vi "Template - P-C StartStop.vi"(7 "Selector":enum16{"Start C-P ", "Clear C-P"}(ring), 8 "error in":errorcluster) -> (0 "error out":errorcluster)   [LabVIEW 2012]
uses:
  Navistar Library/Controls/TypeDef - UEvent Selector(Standard).ctl
  Navistar Library/Controls/TypeDef - Queue Selector(Standard).ctl
  Navistar Library/Controls/TypeDef_Error_Command_enum.ctl
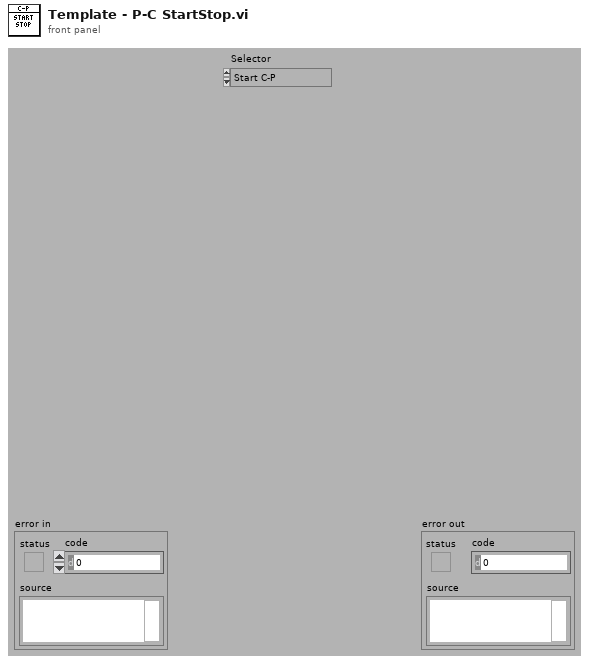
[diagram p1: front panel]
types:
  T1 = typedef "TypeDef_Error_Command_enum.ctl" = enum16{"Init", "Check", "Report"}
  T2 = typedef "TypeDef - UEvent Selector(Standard).ctl" = enum16{"Create UEvent", "Get UEvent Ref", "Clear UEvent", "Reset UEvent", "Generate U Event"}
  T3 = typedef "TypeDef - Queue Selector(Standard).ctl" = enum16{"Create Q", "EnQ", "EnQ at the Opposite", "Flush Q", "Get Q Ref", "Clear Q", "Reset Q"}
  T4 = typedef "TypeDef - Template - UEvent Ref.ctl" = refnum<user-event>
  T5 = typedef "TypeDef - Template - Q1 Ref.ctl" = refnum<queue>
  T6 = typedef "TypeDef - Template - Q2 Ref.ctl" = refnum<queue>
  T7 = cluster{"Q1 Ref":T5, "Q2 Ref":T6, "U-Event Refnum":T4}
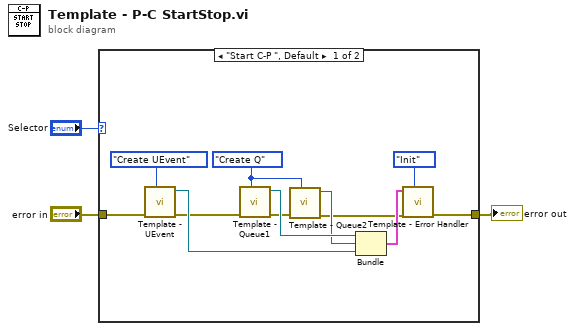
[diagram p0: block diagram]
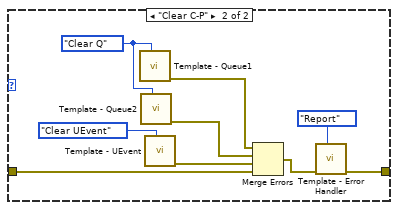
[diagram p2: hidden frame]
diagram:
  n1 = case shown="\"Start C-P \", Default" "Selector" {
    tunnel: "error in" -> [w6 w24]
    tunnel: [w14 w19] -> w2
    frame "Start C-P ", Default {
      w10 = TypeDef_-_Queue_Selector(Standard)."Create Q" ("Queue Selector")
      n2 = call "Template - UEvent.vi"("Event Selector"=TypeDef_-_UEvent_Selector(Standard)."Create UEvent", "error in (no error)"=w6) -> ("error out"=w5:errorcluster, "U-Event Refnum"=w8:T4)  [unwired: 7 in, 1 out]
      n3 = call "Template - Queue1.vi"("Queue Selector"=w10, "error in (no error)"=w5) -> ("error out"=w11:errorcluster, "Q1 Ref"=w12:T5)  [unwired: 7 in, 1 out]
      n4 = call "Template - Queue2.vi"("Queue Selector"=w10, "error in (no error)"=w11) -> ("error out"=w4:errorcluster, "Q2 Ref"=w9:T6)  [unwired: 7 in, 1 out]
      n5 = Bundle("Q1 Ref"=w12, "Q2 Ref"=w9, "U-Event Refnum"=w8) -> (w7:T7)  [unwired: 1 in]
      n6 = call "Template - Error Handler.vi"("Command (Check for Error)"=TypeDef_Error_Command_enum."Init", "error in (no error)"=w4, "QU Ref cluster"=w7) -> ("error out"=w14:errorcluster)  [unwired: 8 in]
    }
    frame "Clear C-P" {
      w17 = TypeDef_-_Queue_Selector(Standard)."Clear Q" ("Queue Selector")
      n7 = call "Template - Queue1.vi"("Queue Selector"=w17) -> ("error out"=w22:errorcluster)  [unwired: 8 in, 2 out]
      n8 = call "Template - Queue2.vi"("Queue Selector"=w17) -> ("error out"=w16:errorcluster)  [unwired: 8 in, 2 out]
      n9 = call "Template - UEvent.vi"("Event Selector"=TypeDef_-_UEvent_Selector(Standard)."Clear UEvent") -> ("error out"=w23:errorcluster)  [unwired: 8 in, 2 out]
      n10 = Merge Errors(w22, w16, w23, w24) -> (w20:errorcluster)
      n11 = call "Template - Error Handler.vi"("Command (Check for Error)"=TypeDef_Error_Command_enum."Report", "error in (no error)"=w20) -> ("error out"=w19:errorcluster)  [unwired: 9 in]
    }
  }
  "error out" <- w2
